vi "Enable-Disable Output.vi"(11 "Enable":bool=TRUE) -> (3 "error out":errorcluster)   [LabVIEW 2014]
doc: "This VI enable or disable the Digital output 11 to 23.\nEnable default is true"
uses:
  <vilib>/rvi/eio/common/nirviEmuTemplateMethod_errors.vi
  <vilib>/eio/EIOMethodNode/EIOMethodNode.xnode
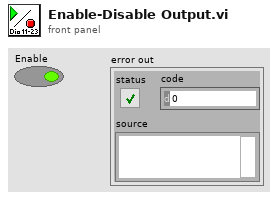
[diagram p1: front panel]
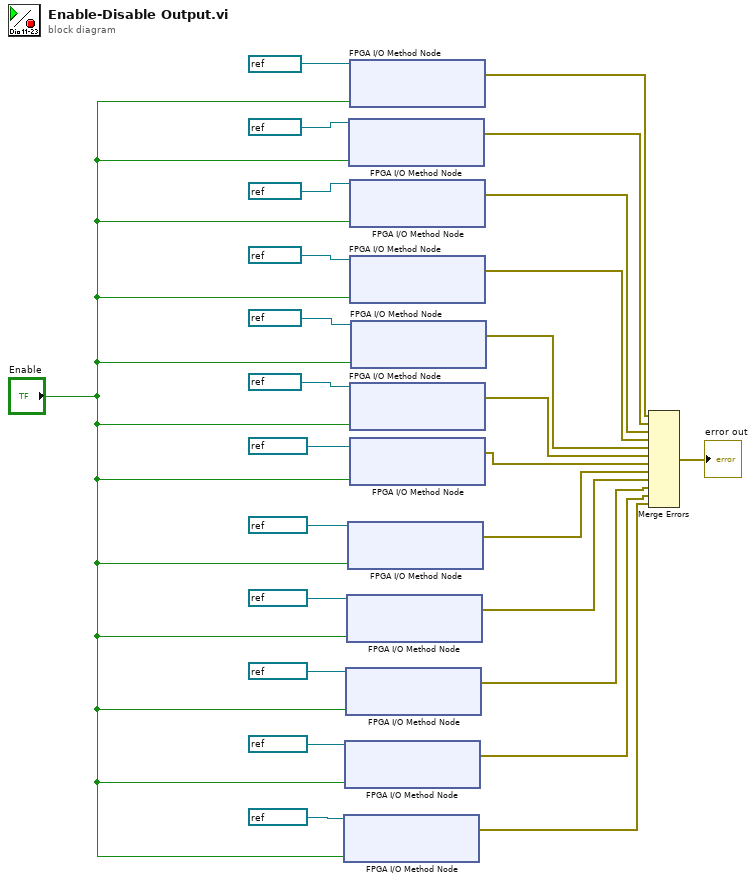
[diagram p0: block diagram]
diagram:
  n1 = xnode "FPGA I/O Method Node"("FPGA I/O In"=refnum<k21> "DIO15", "Enable"="Enable") -> ("error out"=w2:errorcluster)  [unwired: 1 in, 1 out]
  n2 = xnode "FPGA I/O Method Node"("FPGA I/O In"=refnum<k21> "DIO14", "Enable"="Enable") -> ("error out"=w3:errorcluster)  [unwired: 1 in, 1 out]
  n3 = xnode "FPGA I/O Method Node"("FPGA I/O In"=refnum<k21> "DIO13", "Enable"="Enable") -> ("error out"=w4:errorcluster)  [unwired: 1 in, 1 out]
  n4 = xnode "FPGA I/O Method Node"("FPGA I/O In"=refnum<k21> "DIO12", "Enable"="Enable") -> ("error out"=w5:errorcluster)  [unwired: 1 in, 1 out]
  n5 = xnode "FPGA I/O Method Node"("FPGA I/O In"=refnum<k21> "DIO11", "Enable"="Enable") -> ("error out"=w6:errorcluster)  [unwired: 1 in, 1 out]
  n6 = xnode "FPGA I/O Method Node"("FPGA I/O In"=refnum<k21> "DIO5", "Enable"="Enable") -> ("error out"=w12:errorcluster)  [unwired: 1 in, 1 out]
  n7 = xnode "FPGA I/O Method Node"("FPGA I/O In"=refnum<k21> "DIO4", "Enable"="Enable") -> ("error out"=w13:errorcluster)  [unwired: 1 in, 1 out]
  n8 = xnode "FPGA I/O Method Node"("FPGA I/O In"=refnum<k21> "DIO6", "Enable"="Enable") -> ("error out"=w11:errorcluster)  [unwired: 1 in, 1 out]
  n9 = xnode "FPGA I/O Method Node"("FPGA I/O In"=refnum<k21> "DIO7", "Enable"="Enable") -> ("error out"=w10:errorcluster)  [unwired: 1 in, 1 out]
  n10 = xnode "FPGA I/O Method Node"("FPGA I/O In"=refnum<k21> "DIO9", "Enable"="Enable") -> ("error out"=w8:errorcluster)  [unwired: 1 in, 1 out]
  n11 = xnode "FPGA I/O Method Node"("FPGA I/O In"=refnum<k21> "DIO10", "Enable"="Enable") -> ("error out"=w7:errorcluster)  [unwired: 1 in, 1 out]
  n12 = xnode "FPGA I/O Method Node"("FPGA I/O In"=refnum<k21> "DIO8", "Enable"="Enable") -> ("error out"=w9:errorcluster)  [unwired: 1 in, 1 out]
  n13 = Merge Errors(w13, w12, w11, w10, w9, w8, w7, w6, w5, w4, w3, w2) -> (→"error out":errorcluster)
